vi "Initialize.vi"(0 "VISA resource name":refnum<visa-resource-name>, 1 "ID Query? (T: Check)":bool=TRUE, 2 "Reset? (T: Reset)":bool=TRUE, 5 "error in (no error)":errorcluster) -> (14 "VISA resource name out":refnum<visa-resource-name>, 19 "error out":errorcluster)   [LabVIEW 2016, in "Keithley 2000.lvlib"]
doc: "This VI passes the addressing information in the instrument decriptor to the Instr Open VI and returns the instrument ID. You can optionally reset the instrument by setting the front panel reset control. You must run this VI before using any of the instrument driver VIs for this instrument.\n\nNote:\nIf you wish to use the serial interface, set the serial settings on the instrument to be the same as the serial settings on the block diagram. If you have problems with serial settings and the instrument is configured with the same serial settings as the block diagram, try lowering the baud rate (on both the instrument and on the block diagram)."
uses:
  Keithley 2000.lvlib
panel:
  # "© 2003, National Instruments, Corporation.  All Rights Reserved."
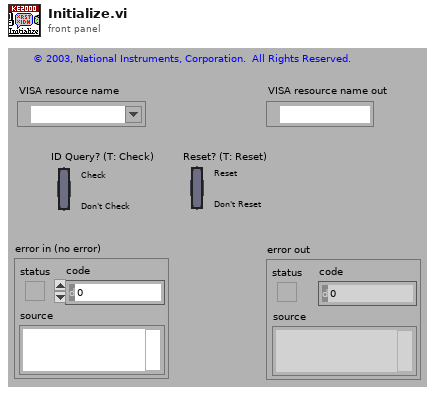
[diagram p1: front panel]
types:
  T1 = cluster{"Status":bool, "Code":i32, "Source (VI Name)":string}
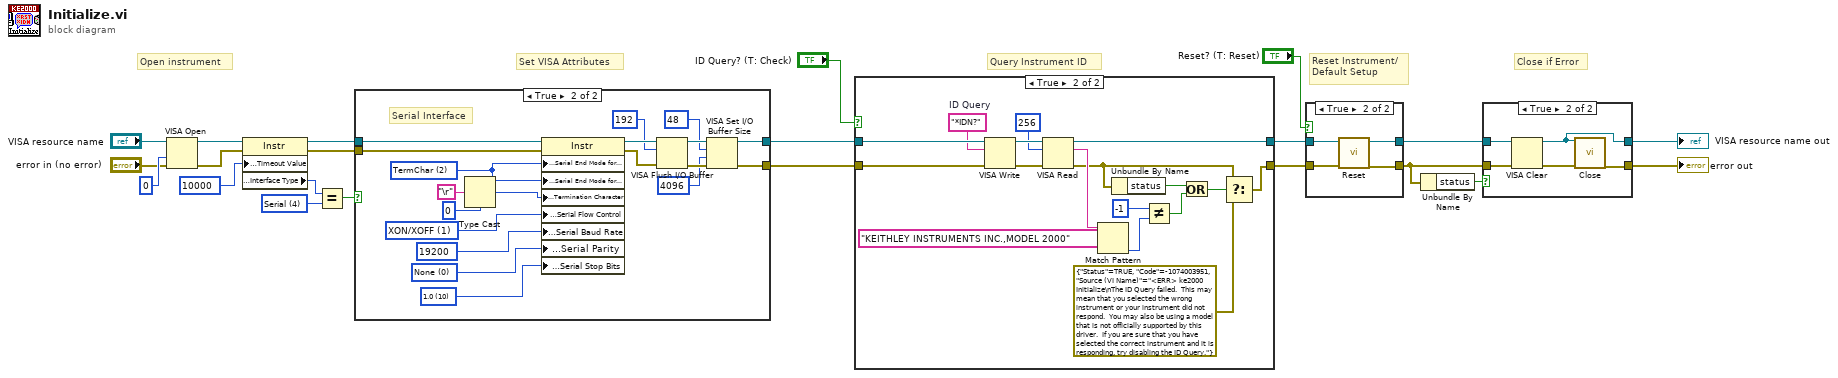
[diagram p0: block diagram]
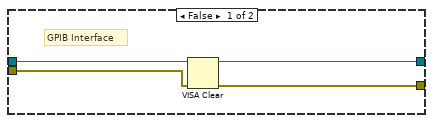
[diagram p2: hidden frame]
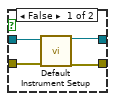
[diagram p4: hidden frame]
diagram:
  w8 = u16 4 items=["GPIB"=1, "VXI"=2, "GPIB-VXI"=3, "Serial"=4, "PXI"=5, "TCPIP"=6, "USB"=7] ("Interface Information:Interface Type")
  # "Set VISA Attributes"
  # "Close if Error"
  # "Query Instrument ID"
  # "Reset Instrument/\nDefault Setup"
  # "Open instrument"
  n1 = VISA Open(access mode=u32 0, error in (no error)="error in (no error)", VISA resource name="VISA resource name") -> (VISA resource name=w4:refnum<visa-resource-name>, error out=w3:errorcluster)  [unwired: 2 in]
  n2 = property class="Instr"(reference=w4, error in=w3, "General Settings:Timeout Value"=u32 10000) -> (reference out=w11:refnum<visa-resource-name>, error out=w10:errorcluster, "Interface Information:Interface Type"=w15:u16)
  n3 = Equal?(x=w15, y=w8) -> (x = y?=w9:bool)
  n4 = case shown="True" w9 {
    tunnel: [w24 w42] -> w13
    tunnel: [w23 w39] -> w12
    tunnel: w11 -> [w26 w44]
    tunnel: w10 -> [w25 w45]
    frame False {
      # "GPIB Interface"
      n5 = VISA Clear(VISA resource name=w26, error in (no error)=w25) -> (VISA resource name out=w24:refnum<visa-resource-name>, error out=w23:errorcluster)
    }
    frame True {
      w27 = u16 10 items=["1.0"=10, "1.5"=15, "2.0"=20] ("Serial Settings:Serial Stop Bits")
      w30 = u16 0 items=["None", "Odd", "Even", "Mark", "Space"] ("Serial Settings:Serial Parity")
      w32 = u16 2 items=["None", "LastBit", "TermChar"] ("Serial Settings:Serial End Mode for Reads")
      w28 = u16 1 items=["None"=0, "XON/XOFF"=1, "RTS/CTS"=2, "DTR/DSR"=4] ("Serial Settings:Serial Flow Control")
      # "Serial Interface"
      n6 = Type Cast(type=u8 0, x="\r") -> (*(type *) &x=w31:u8)
      n7 = property class="Instr"(reference=w44, error in=w45, "Serial Settings:Serial End Mode for Reads"=w32, "Serial Settings:Serial End Mode for Writes"=w32, "Message Based Settings:Termination Character"=w31, "Serial Settings:Serial Flow Control"=w28, "Serial Settings:Serial Baud Rate"=u32 19200, "Serial Settings:Serial Parity"=w30, "Serial Settings:Serial Stop Bits"=w27) -> (reference out=w38:refnum<visa-resource-name>, error out=w41:errorcluster)
      n8 = VISA Flush I/O Buffer(VISA resource name=w38, mask (16)=u16 192, error in (no error)=w41) -> (VISA resource name out=w43:refnum<visa-resource-name>, error out=w40:errorcluster)
      n9 = VISA Set I/O Buffer Size(VISA resource name=w43, mask (16)=u16 48, size (4096)=u32 4096 ("size (0)"), error in (no error)=w40) -> (VISA resource name out=w42:refnum<visa-resource-name>, error out=w39:errorcluster)
    }
  }
  n10 = case shown="True" "ID Query? (T: Check)" {
    tunnel: [w46 w64] -> w21
    tunnel: [w47 w61] -> w22
    tunnel: w13 -> [w47 w62]
    tunnel: w12 -> [w46 w63]
    frame False {
    }
    frame True {
      w49 = "*IDN?"  # ID Query
      n11 = VISA Write(VISA resource name=w62, write buffer=w49, error in (no error)=w63) -> (VISA resource name out=w58:refnum<visa-resource-name>, error out=w56:errorcluster)  [unwired: 1 out]
      n12 = VISA Read(VISA resource name=w58, byte count=u32 256, error in (no error)=w56) -> (VISA resource name out=w61:refnum<visa-resource-name>, read buffer=w59:string, error out=w57:errorcluster)  [unwired: 1 out]
      n13 = Match Pattern(string=w59, regular expression="KEITHLEY INSTRUMENTS INC.,MODEL 2000") -> (offset past match=w51:i32)  [unwired: 1 in, 3 out]
      n14 = Unbundle By Name(w57) -> ("status"=w54:bool)
      n15 = Not Equal?(x=-1, y=w51) -> (x != y?=w60:bool)
      n16 = Or(x=w54, y=w60) -> (x .or. y?=w55:bool)
      n17 = Select(t=w57, s=w55, f=T1 {"Status"=TRUE, "Code"=-1074003951, "Source (VI Name)"="<ERR> ke2000 Initialize\nThe ID Query failed.  This may mean that you selected the wrong instrument or your instrument did not respond.  You may also be using a model that is not officially supported by this driver.  If you are sure that you have selected the correct instrument and it is responding, try disabling the ID Query."}) -> (s? t:f=w64:T1)
    }
  }
  n18 = case shown="True" "Reset? (T: Reset)" {
    tunnel: w21 -> [w65 w69]
    tunnel: [w66 w72] -> w6
    tunnel: w22 -> [w68 w70]
    tunnel: [w67 w71] -> w18
    frame False {
      n19 = call "Default Instrument Setup.vi"("VISA resource name"=w68, "error in (no error)"=w65) -> ("VISA resource name out"=w67:refnum<visa-resource-name>, "error out"=w66:errorcluster)  [unwired: 16 in]
    }
    frame True {
      n20 = call "Reset.vi"("VISA resource name"=w70, "error in (no error)"=w69) -> ("VISA resource name out"=w71:refnum<visa-resource-name>, "error out"=w72:errorcluster)  [unwired: 16 in]
    }
  }
  n21 = Unbundle By Name(w6) -> ("status"=w5:bool)
  n22 = case shown="True" w5 {
    tunnel: w18 -> [w74 w78]
    tunnel: [w74 w77] -> w17
    tunnel: [w73 w79] -> w2
    tunnel: w6 -> [w73 w76]
    frame False {
    }
    frame True {
      n23 = VISA Clear(VISA resource name=w78, error in (no error)=w76) -> (VISA resource name out=w77:refnum<visa-resource-name>, error out=w75:errorcluster)
      n24 = call "Close.vi"("VISA resource name"=w77, "error in (no error)"=w75) -> ("error out"=w79:errorcluster)  [unwired: 17 in]
    }
  }
  "VISA resource name out" <- w17
  "error out" <- w2
